vi "Refresh_Image.vi"() -> ()   [LabVIEW 2012]
uses:
  AUTO_GUIDER.llb/Webcam depth.ctl
  Global_Telescopio.vi
  AUTO_GUIDER.llb/Global_Mao.vi
  <vilib>/vision/NI_Vision_Development_Module.lvlib
panel:
  in  "Case Constant\n(See Context Help)":bool
  out "Imagem Saída":picture
  out "Draw Area Size":cluster{"Width":u32, "Height":u32}
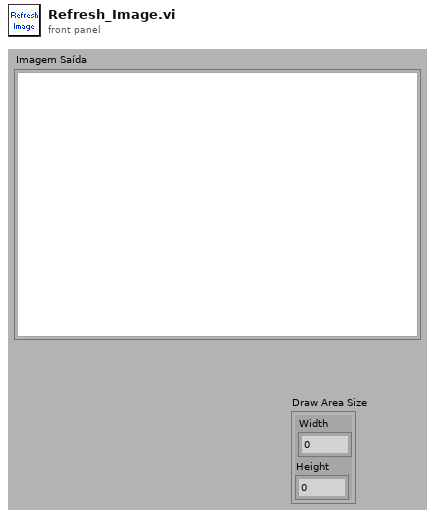
[diagram p1: front panel]
types:
  T1 = typedef "Webcam depth.ctl" = enum16{"24-bit", "8-bit"}
  T2 = cluster{"bit depth":u8, "rect":cluster{"left":i16, "top":i16, "right":i16, "bottom":i16}, "Initialized image array":u8[][], "color table":u32[]}
  T3 = typedef "IMAQ Image.ctl" = refnum<image>
  T4 = typedef "Webcam rect.ctl" = cluster{"left":i16, "top":i16, "right":i16, "bottom":i16}
  T5 = cluster{"left":i16, "top":i16, "right":i16, "bottom":i16}
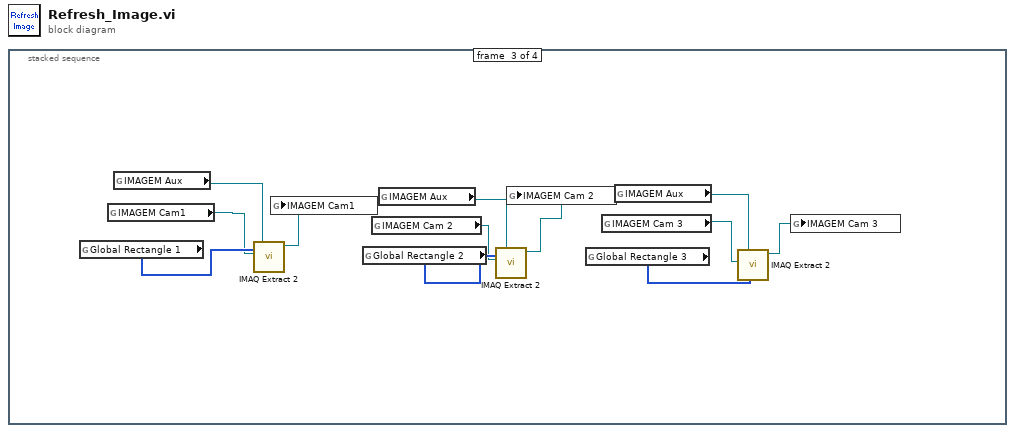
[diagram p0: block diagram]
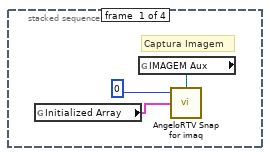
[diagram p2: hidden frame]
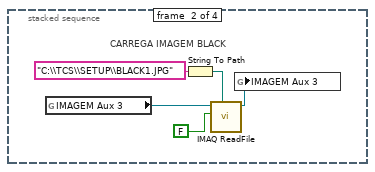
[diagram p3: hidden frame]
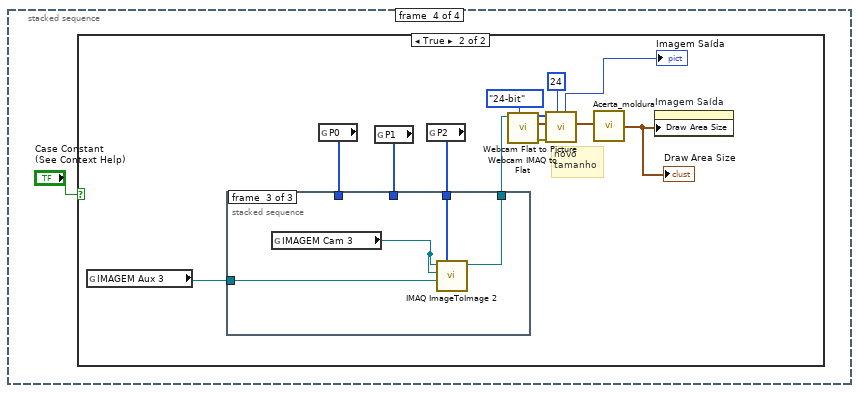
[diagram p4: hidden frame]
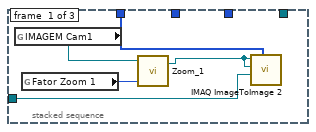
[diagram p6: hidden frame]
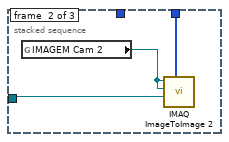
[diagram p7: hidden frame]
diagram:
  n1 = stacked-sequence {
    frame #0 {
      # "Captura Imagem"
      n2 = global read "Global_Telescopio.vi" "Initialized Array"() -> (w2:T2)
      n3 = global read "Global_Mao.vi" "IMAGEM Aux"() -> (w1:T3)
      n4 = call "AngeloRTV Snap for imaq.vi"("Image In"=w1, "Initialized Array"=w2, "PortNo"=u16 0) -> ()  [unwired: 1 in, 2 out]
    }
    frame #1 {
      # "CARREGA IMAGEM BLACK"
      n5 = global read "Global_Mao.vi" "IMAGEM Aux 3"() -> (w4:T3)
      n6 = String To Path(string="C:\\TCS\\SETUP\\BLACK1.JPG" ("SOMENTE DIRETORIO")) -> (path=w8:path)
      n7 = call "IMAQ ReadFile"("File Path"=w8, "Load Color Palette? (No)"=FALSE, "Image"=w4) -> ("Image Out"=w5:T3)  [unwired: 4 in, 4 out]
      n8 = global write "Global_Mao.vi" "IMAGEM Aux 3"(w5) -> ()
    }
    frame #2 {
      n9 = global read "Global_Telescopio.vi" "Global Rectangle 1"() -> (w20:i32[])
      n10 = global read "Global_Mao.vi" "IMAGEM Cam1"() -> (w14:T3)
      n11 = global read "Global_Mao.vi" "IMAGEM Aux"() -> (w16:T3)
      n12 = call "IMAQ Extract 2"("Optional Rectangle"=w20, "Image Dst"=w14, "Image Src"=w16) -> ("Image Dst Out"=w15:T3)  [unwired: 7 in, 1 out]
      n13 = global write "Global_Mao.vi" "IMAGEM Cam1"(w15) -> ()
      n14 = global read "Global_Telescopio.vi" "Global Rectangle 2"() -> (w19:i32[])
      n15 = global read "Global_Mao.vi" "IMAGEM Cam 2"() -> (w11:T3)
      n16 = global read "Global_Mao.vi" "IMAGEM Aux"() -> (w17:T3)
      n17 = call "IMAQ Extract 2"("Optional Rectangle"=w19, "Image Dst"=w11, "Image Src"=w17) -> ("Image Dst Out"=w12:T3)  [unwired: 7 in, 1 out]
      n18 = global write "Global_Mao.vi" "IMAGEM Cam 2"(w12) -> ()
      n19 = global read "Global_Telescopio.vi" "Global Rectangle 3"() -> (w18:i32[])
      n20 = global read "Global_Mao.vi" "IMAGEM Cam 3"() -> (w10:T3)
      n21 = global read "Global_Mao.vi" "IMAGEM Aux"() -> (w13:T3)
      n22 = call "IMAQ Extract 2"("Optional Rectangle"=w18, "Image Dst"=w10, "Image Src"=w13) -> ("Image Dst Out"=w9:T3)  [unwired: 7 in, 1 out]
      n23 = global write "Global_Mao.vi" "IMAGEM Cam 3"(w9) -> ()
    }
    frame #3 {
      n24 = case shown="True" "Case Constant\n(See Context Help)" {
        frame False {
        }
        frame True {
          # "novo\ntamanho"
          n25 = global read "Global_Mao.vi" "IMAGEM Aux 3"() -> (w23:T3)
          n26 = global read "Global_Telescopio.vi" "P0"() -> (w27:i32[])
          n27 = global read "Global_Telescopio.vi" "P1"() -> (w26:i32[])
          n28 = global read "Global_Telescopio.vi" "P2"() -> (w25:i32[])
          n29 = stacked-sequence {
            tunnel: w25 -> [_ _ w46]
            tunnel: [_ _ w45] -> w34
            tunnel: w23 -> [w38 w41 w44]
            tunnel: w26 -> [_ w42 _]
            tunnel: w27 -> [w39 _ _]
            frame #0 {
              n30 = global read "Global_Mao.vi" "IMAGEM Cam1"() -> (w37:T3)
              n31 = global read "Global_Telescopio.vi" "Fator Zoom 1"() -> (w36:i32)
              n32 = call "Zoom_1.vi"("Fator Zoom"=w36, "IMAGEM Cam1"=w37) -> ("Image Dst Out 2"=w35:T3)  [unwired: 2 in]
              n33 = call "IMAQ ImageToImage 2"("Offset Left/Top"=w39, "Image Dst"=w38, "Image Src (Small)"=w35, "Image Src (Large)"=w35) -> ()  [unwired: 6 in, 2 out]
            }
            frame #1 {
              n34 = global read "Global_Mao.vi" "IMAGEM Cam 2"() -> (w40:T3)
              n35 = call "IMAQ ImageToImage 2"("Offset Left/Top"=w42, "Image Dst"=w41, "Image Src (Small)"=w40, "Image Src (Large)"=w40) -> ()  [unwired: 6 in, 2 out]
            }
            frame #2 {
              n36 = global read "Global_Mao.vi" "IMAGEM Cam 3"() -> (w43:T3)
              n37 = call "IMAQ ImageToImage 2"("Offset Left/Top"=w46, "Image Dst"=w44, "Image Src (Small)"=w43, "Image Src (Large)"=w43) -> ("Image Dst Out"=w45:T3)  [unwired: 6 in, 1 out]
            }
          }
          n38 = call "Webcam IMAQ to Flat.vi"("depth (8)"=Webcam_depth."24-bit", "Image"=w34) -> ("error out"=w29:errorcluster, "rect"=w30:T4, "flat image"=w31:u8[])  [unwired: 5 in]
          n39 = call "Webcam Flat to Picture.vi"("depth 24/8"=u8 24, "error in"=w29, "rect in"=w30, "flat image in"=w31) -> ("rect out"=w32:T5, "picture"=→"Imagem Saída":picture)  [unwired: 3 in, 2 out]
          n40 = call "Acerta_moldura.vi"("input cluster"=w32) -> ("Draw Area Size"=w33:cluster{"Width":u32, "Height":u32})  [unwired: 4 in]
          "Draw Area Size" <- w33
          n41 = property on="Imagem Saída" class="Pict"("Draw Area Size"=w33) -> ()  [unwired: 2 in, 2 out]
        }
      }
    }
  }
